vi "Test.vi"() -> ()   [LabVIEW 2019]
uses:
  Sensors/Detector/Event.ctl
  Sensors/Arduino/Arduino Detector.lvclass
  C:/LabVIEW Sources/Muon Detector/Sensors/Detector/Muon Detector.lvclass
  Sensors/Arduino/Arduino Detector.lvclass/Arduino Detector.ctl
  Sensors/Simulated/Simulated Detector.lvclass
  Sensors/Detector/Muon Detector.lvclass
panel:
  out "Event":T1
  out "Waveform Chart":i32(graph)
  out "error out":errorcluster
  out "Name":string
  in  "Stop":bool
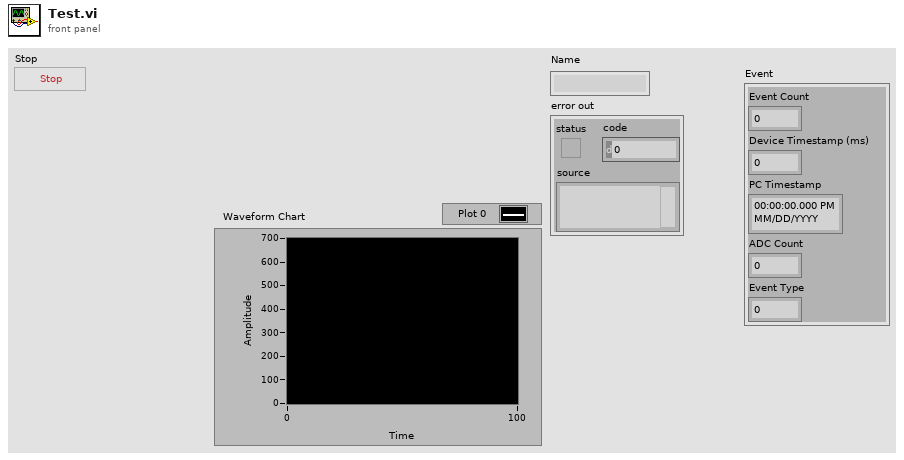
[diagram p1: front panel]
types:
  T1 = typedef "Muon Detector.lvclass/Event.ctl" = cluster{"Event Count":i32, "Device Timestamp (ms)":i32, "PC Timestamp":timestamp, "ADC Count":i32, "Event Type":u8}
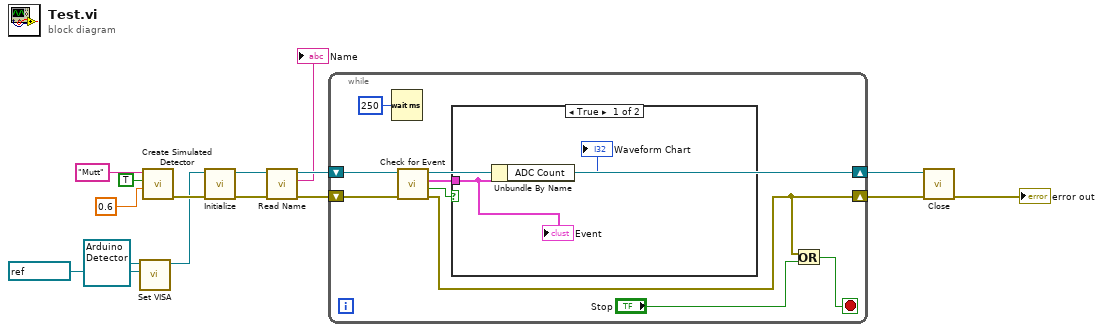
[diagram p0: block diagram]
diagram:
  n1 = call "Set VISA.vi"("VISA"=refnum<visa-resource-name> "COM5", "Arduino Detector in"=refnum<class "Arduino Detector.lvclass"> refnum) -> ("Arduino Detector out"=w3:refnum<class "Arduino Detector.lvclass">)  [unwired: 8 in, 1 out]
  n2 = call "Create Simulated Detector.vi"("Event Threshold (0-1)"=0.6 ("y"), "Master"=TRUE, "Name"="Mutt") -> ("error out"=w15:errorcluster)  [unwired: 7 in, 1 out]
  n3 = call-dynamic "Initialize.vi"("error in (no error)"=w15, "Arduino Detector in"=w3) -> ("error out"=w13:errorcluster, "Arduino Detector out"=w14:refnum<class "Arduino Detector.lvclass">)  [unwired: 8 in]
  n4 = call-dynamic "Read Name.vi"("error in (no error)"=w13, "Arduino Detector in"=w14) -> ("error out"=w11:errorcluster, "Name"=→"Name":string, "Arduino Detector out"=w12:refnum<class "Arduino Detector.lvclass">)  [unwired: 7 in]
  n5 = while {
    shift-right: [w22] -> w10
    shift-left: w12 -> [w24]
    shift-right: [w18] -> w9
    shift-left: w11 -> [w23]
    stop <- w19 stop-if-true
    n6 = Wait (ms)(milliseconds to wait=u32 250) -> ()  [unwired: 1 out]
    n7 = call "Check for Event.vi"("error in (no error)"=w23, "Muon Detector in"=w24) -> ("error out"=w18:errorcluster, "Valid?"=w17:bool, "Event"=w16:T1, "Muon Detector out"=w22:refnum<class "Arduino Detector.lvclass">)  [unwired: 6 in]
    n8 = case shown="True" w17 {
      tunnel: w16 -> [w25 _]
      frame True {
        n9 = Unbundle By Name(w25) -> ("ADC Count"=→"Waveform Chart":i32)
        "Event" <- w25
      }
      frame False {
      }
    }
    n10 = Or(x=w18, y="Stop") -> (x .or. y?=w19:bool)
  }
  n11 = call-dynamic "Close.vi"("error in (no error)"=w9, "Arduino Detector in"=w10) -> ("error out"=→"error out":errorcluster)  [unwired: 8 in, 1 out]
